vi "Num of Colors to Color Array.vi"(4 "# of Colors":i32=5, 5 "Color Array Type":T1(ring)) -> (1 "Colors Array":u32[](array[colorbox])=[16711680, 13434624, 65382, 26111, 13435135])   [LabVIEW 2010]
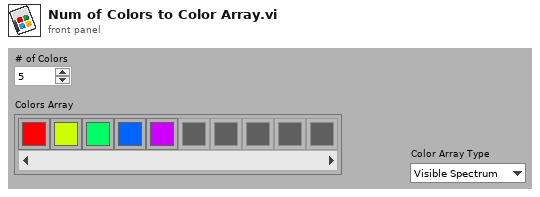
[diagram p1: front panel]
types:
  T1 = enum16{"Visible Spectrum", "Greyscale", "Contrasting Colors"}
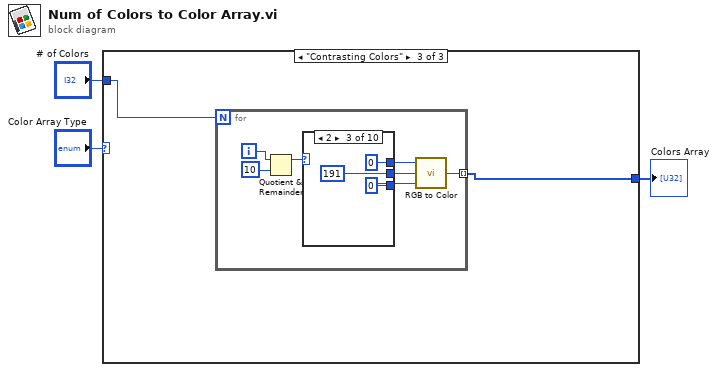
[diagram p0: block diagram]
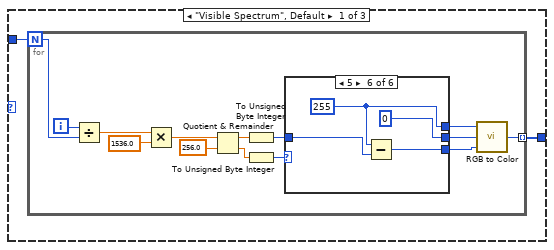
[diagram p2: hidden frame]
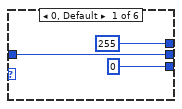
[diagram p3: hidden frame]
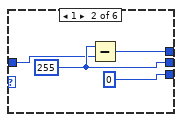
[diagram p4: hidden frame]
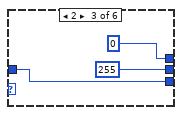
[diagram p5: hidden frame]
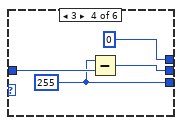
[diagram p6: hidden frame]
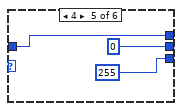
[diagram p7: hidden frame]
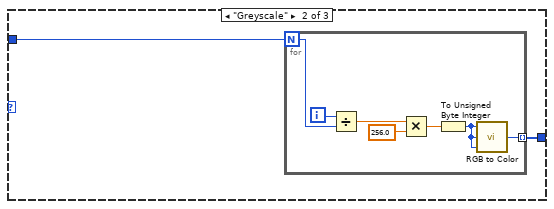
[diagram p8: hidden frame]
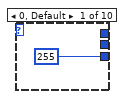
[diagram p9: hidden frame]
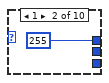
[diagram p10: hidden frame]
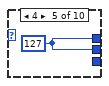
[diagram p12: hidden frame]
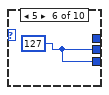
[diagram p13: hidden frame]
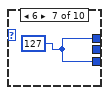
[diagram p14: hidden frame]
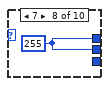
[diagram p15: hidden frame]
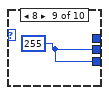
[diagram p16: hidden frame]
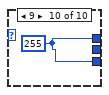
[diagram p17: hidden frame]
diagram:
  n1 = case shown="\"Contrasting Colors\"" "Color Array Type" {
    tunnel: [w5 w42 w50] -> w3
    tunnel: "# of Colors" -> [w4 w41 w51]
    frame "Visible Spectrum", Default {
      n2 = for {
        N: w4 -> [w19]
        tunnel: [w14] -> w5 mode=indexing
        i -> [w6]
        n3 = Divide(x=w6, y=w19) -> (x/y=w17:dbl)
        n4 = Multiply(x=w17, y=1536.0) -> (x*y=w15:dbl)
        n5 = Quotient & Remainder(x=w15, y=256.0) -> (x-y*floor(x/y)=w13:dbl, floor(x/y)=w12:dbl)
        n6 = To Unsigned Byte Integer(number=w13) -> (unsigned 8bit integer=w10:u8)
        n7 = To Unsigned Byte Integer(number=w12) -> (unsigned 8bit integer=w11:u8)
        n8 = case shown="5" w11 {
          tunnel: w10 -> [w21 w24 w27 w32 w35 w38]
          tunnel: [u8 255 ("R") w23 u8 0 ("R") u8 0 ("R") w35 w39] -> w9
          tunnel: [w21 w25 u8 255 ("R") w31 u8 0 ("R") u8 0 ("R")] -> w8
          tunnel: [u8 0 ("R") u8 0 ("R") w27 w30 u8 255 ("R") w37] -> w7
          frame 0, Default {
          }
          frame 1 {
            w25 = u8 255 ("R")
            n9 = Subtract(x=w25, y=w24) -> (x-y=w23:u8)
          }
          frame 2 {
          }
          frame 3 {
            w30 = u8 255 ("R")
            n10 = Subtract(x=w30, y=w32) -> (x-y=w31:u8)
          }
          frame 4 {
          }
          frame 5 {
            w39 = u8 255 ("R")
            n11 = Subtract(x=w39, y=w38) -> (x-y=w37:u8)
          }
        }
        n12 = call <vilib>:"RGB to Color.vi"("B"=w7, "G"=w8, "R"=w9) -> ("Color"=w14:u32)
      }
    }
    frame "Greyscale" {
      n13 = for {
        N: w41 -> [w49]
        tunnel: [w46] -> w42 mode=indexing
        i -> [w45]
        n14 = Divide(x=w45, y=w49) -> (x/y=w48:dbl)
        n15 = Multiply(x=w48, y=256.0) -> (x*y=w44:dbl)
        n16 = To Unsigned Byte Integer(number=w44) -> (unsigned 8bit integer=w43:u8)
        n17 = call <vilib>:"RGB to Color.vi"("B"=w43, "G"=w43, "R"=w43) -> ("Color"=w46:u32)
      }
    }
    frame "Contrasting Colors" {
      n18 = for {
        N: w51 -> [_]
        tunnel: [w52] -> w50 mode=indexing
        i -> [w58]
        n19 = Quotient & Remainder(x=w58, y=10) -> (x-y*floor(x/y)=w56:i32)  [unwired: 1 out]
        n20 = case shown="2" w56 {
          tunnel: [255 _ 0 _ _ w65 w66 _ w68 w69] -> w55
          tunnel: [_ 255 0 _ w64 _ w66 w67 _ w69] -> w54
          tunnel: [_ _ 191 _ w64 w65 _ w67 w68 _] -> w53
          frame 0, Default {
          }
          frame 1 {
          }
          frame 2 {
          }
          frame 3 {
          }
          frame 4 {
            w64 = 127
          }
          frame 5 {
            w65 = 127
          }
          frame 6 {
            w66 = 127
          }
          frame 7 {
            w67 = 255
          }
          frame 8 {
            w68 = 255
          }
          frame 9 {
            w69 = 255
          }
        }
        n21 = call <vilib>:"RGB to Color.vi"("B"=w55, "G"=w53, "R"=w54) -> ("Color"=w52:u32)
      }
    }
  }
  "Colors Array" <- w3
